vi "Control Init.vi"(7 "VolatusAPI":refnum<class "VolatusAPI.lvclass">, 8 "error in (no error)":errorcluster, 10 "JSON":string, 11 "2WayValve in":refnum<class "2WayValveH.lvclass">) -> (0 "error out":errorcluster, 3 "2WayValve out":refnum<class "2WayValveH.lvclass">)   [LabVIEW 2020, in "VolatusGUIElements.lvlib" / "2WayValveH.lvclass"]
uses:
  2WayValveH.lvclass
  2WayValveH.lvclass/2WayValveH.ctl
  5ca493e1-1c63-4061-b4b4-46184d61fbe0.vi
  Group Channel.ctl
  JSON.ctl
  Unused Element.ctl
  Volatus/VolatusAPI/VolatusAPI.lvclass
  lv-vecto/Vecto/Group/Group.lvclass
  Channel State.ctl
  Values.ctl
  C:/dev/lv20CE/relink/lv-vecto/Vecto/GroupAbstract/GroupAbstract.lvclass
  C:/dev/lv20CE/relink/lv-vecto/Vecto/Group/Group.lvclass
  lv-vecto/Vecto/Channel/Channel.lvclass
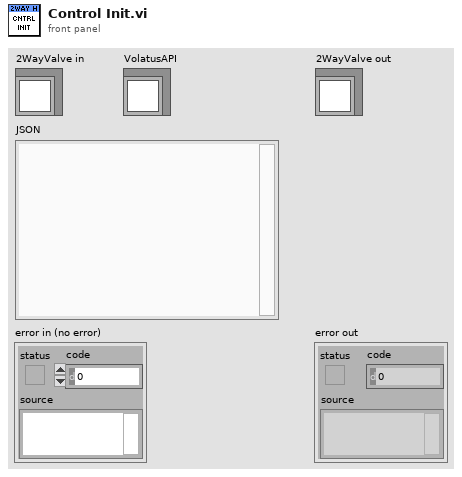
[diagram p1: front panel]
types:
  T1 = typedef "VolatusGUIElements.lvlib/2WayValveH.lvclass/Values.ctl" = cluster{"Command":T2, "CmdFB":T2, "Closed":T2, "Open":T2, "Energized":T2}
  T2 = typedef "VolatusGUIElements.lvlib/2WayValveH.lvclass/Channel State.ctl" = cluster{"Value":bool, "Stale":bool, "Config":bool, "Error":bool, "Prev":bool}
  T3 = typedef "VolatusGUIElements.lvlib/2WayValveH.lvclass/Unused Element.ctl" = cluster{"Command":bool, "Feedback":bool, "Energized":bool}
  T4 = typedef "VolatusGUIElements.lvlib/2WayValveH.lvclass/JSON.ctl" = cluster{"Output":T5, "ClosedFB":T5, "OpenFB":T5, "Energized":T5, "Staleness":dbl}
  T5 = typedef "VolatusGUIElements.lvlib/2WayValveH.lvclass/Group Channel.ctl" = cluster{"Channel":string}
  T6 = typedef "VectoConfig.lvlib/Channel Info.ctl" = cluster{"Name":string, "Group":string, "Owning Node":string, "Owning Task":string, "Resource":string}
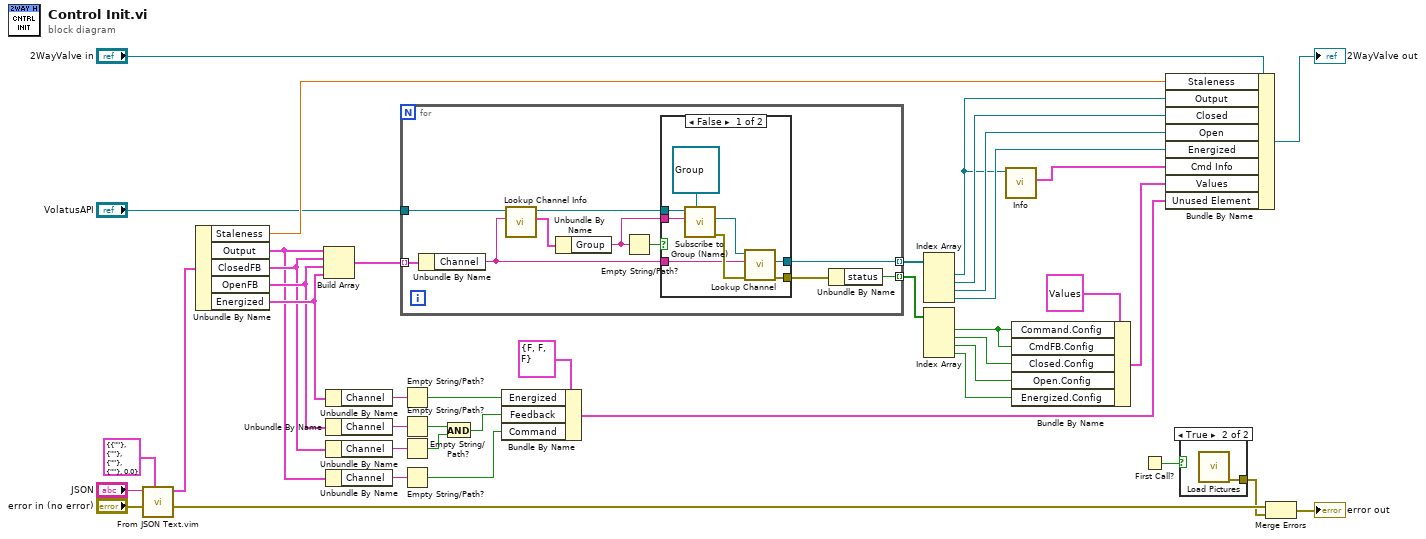
[diagram p0: block diagram]
diagram:
  n1 = call "From JSON Text.vim"("Data Type and Default Value"=T4 {"Output"={"Channel"=""}, "ClosedFB"={"Channel"=""}, "OpenFB"={"Channel"=""}, "Energized"={"Channel"=""}, "Staleness"=0.0} ("JSON"), "error in (no error)"="error in (no error)", "JSON"="JSON") -> ("error out"=w38:errorcluster, "Data out"=w37:T4)  [unwired: 7 in]
  n2 = Unbundle By Name(w37) -> ("Staleness"=w8:dbl, "Output"=w3:T5, "ClosedFB"=w34:T5, "OpenFB"=w35:T5, "Energized"=w36:T5)
  n3 = Build Array(w3, w34, w35, w36) -> (w23:T5[])
  n4 = Unbundle By Name(w36) -> ("Channel"=w33:string)
  n5 = Unbundle By Name(w35) -> ("Channel"=w32:string)
  n6 = Unbundle By Name(w34) -> ("Channel"=w31:string)
  n7 = Unbundle By Name(w3) -> ("Channel"=w30:string)
  n8 = for {
    tunnel: w23 -> [w50] mode=indexing
    tunnel: [w49] -> w22 mode=indexing
    tunnel: [w47] -> w21 mode=indexing
    tunnel: "VolatusAPI" -> [w51]
    n9 = Unbundle By Name(w50) -> ("Channel"=w44:string)
    n10 = call "Lookup Channel Info.vi"("Channel Name"=w44, "VolatusAPI in"=w51) -> ("Channel Info"=w43:T6, "VolatusAPI out"=w45:refnum<class "VolatusAPI.lvclass">)  [unwired: 6 in, 2 out]
    n11 = Unbundle By Name(w43) -> ("Group"=w42:string)
    n12 = Empty String/Path?(string/path=w42) -> (empty?=w46:bool)
    n13 = case shown="False" w46 {
      tunnel: w45 -> [w58 _]
      tunnel: w42 -> [w56 _]
      tunnel: w44 -> [w54 _]
      tunnel: [w53 _] -> w49
      tunnel: [w52 _] -> w48
      frame False {
        n14 = call "Subscribe to Group (Name).vi"("Group Type"=refnum<class "Group.lvclass"> refnum ("Vecto.lvlib:Group.lvclass"), "Group Name"=w56, "VolatusAPI in"=w58) -> ("error out"=w59:errorcluster, "Group"=w55:refnum<class "Group.lvclass">)  [unwired: 6 in, 1 out]
        n15 = call "Lookup Channel.vi"("error in (no error)"=w59, "Channel Name"=w54, "Group in"=w55) -> ("error out"=w52:errorcluster, "Channel"=w53:refnum<class "Channel.lvclass">)  [unwired: 6 in, 1 out]
      }
      frame True {
      }
    }
    n16 = Unbundle By Name(w48) -> ("status"=w47:bool)
  }
  n17 = Empty String/Path?(string/path=w33) -> (empty?=w28:bool)
  n18 = Empty String/Path?(string/path=w32) -> (empty?=w27:bool)
  n19 = Empty String/Path?(string/path=w31) -> (empty?=w26:bool)
  n20 = Empty String/Path?(string/path=w30) -> (empty?=w24:bool)
  n21 = And(x=w27, y=w26) -> (x .and. y?=w25:bool)
  n22 = Bundle By Name(cluster=T3 {"Command"=FALSE, "Feedback"=FALSE, "Energized"=FALSE} ("Unused Element"), "Energized"=w28, "Feedback"=w25, "Command"=w24) -> (w11:T3)
  n23 = Index Array(array=w22) -> (element #1=w2:refnum<class "Channel.lvclass">, element #2=w15:refnum<class "Channel.lvclass">, element #3=w14:refnum<class "Channel.lvclass">, element #4=w13:refnum<class "Channel.lvclass">)  [unwired: 4 in]
  n24 = Index Array(array=w21) -> (element #1=w19:bool, element #2=w18:bool, element #3=w17:bool, element #4=w16:bool)  [unwired: 4 in]
  n25 = call "Info.vi"("Channel in"=w2) -> ("Info"=w1:T6)  [unwired: 8 in, 2 out]
  n26 = Bundle By Name(cluster=T1 {"Command"={"Value"=FALSE, "Stale"=FALSE, "Config"=FALSE, "Error"=FALSE, "Prev"=FALSE}, "CmdFB"={"Value"=FALSE, "Stale"=FALSE, "Config"=FALSE, "Error"=FALSE, "Prev"=FALSE}, "Closed"={"Value"=FALSE, "Stale"=FALSE, "Config"=FALSE, "Error"=FALSE, "Prev"=FALSE}, "Open"={"Value"=FALSE, "Stale"=FALSE, "Config"=FALSE, "Error"=FALSE, "Prev"=FALSE}, "Energized"={"Value"=FALSE, "Stale"=FALSE, "Config"=FALSE, "Error"=FALSE, "Prev"=FALSE}} ("Values"), "Command.Config"=w19, "CmdFB.Config"=w19, "Closed.Config"=w18, "Open.Config"=w17, "Energized.Config"=w16) -> (w12:T1)
  n27 = First Call?() -> (First Call?: T/F=w7:bool)
  n28 = Bundle By Name(cluster="2WayValve in", "Staleness"=w8, "Output"=w2, "Closed"=w15, "Open"=w14, "Energized"=w13, "Cmd Info"=w1, "Values"=w12, "Unused Element"=w11) -> (→"2WayValve out":refnum<class "2WayValveH.lvclass">)
  n29 = case shown="True" w7 {
    tunnel: [_ w60] -> w5
    frame False {
    }
    frame True {
      n30 = call "Load Pictures.vi"() -> ("error out"=w60:errorcluster)  [unwired: 11 in]
    }
  }
  n31 = Merge Errors(w38, w5) -> (→"error out":errorcluster)
